vi "Get Menu Items.vi"() -> ()   [LabVIEW 2010]
panel:
  in  "Status 2":string[][](array[string])=[["File: Data Log", "正在进行数据记录"], ["File: Copy Parameters", "正在复制参数"], ["File: Print", "正在打印"], ["File: Export", "正在导出"], ["File: Exit", "退出"], ["Users: Login", "用户登录"], ["Users: Management", "用户管理"], ["System - Comm", "系统通信状态"], ["System: Comm Diags", "系统通信诊断"], ["System: Comm Enable", "通信使能"], ["System: Comm Disable", "通信禁用"], ["System: Snapshot", "系统快照"], ["System: Snapshot Save", "保存快照"], ["System: Snapshot Restore", "恢复快照"], ["System: Snapshot Remove", "删除快照"], ["Recipe: New", "新建Recipe"], ["Recipe: Open", "打开Recipe"], ["Recipe: Save", "保存Recipe"], ["Recipe: Save As", "另存Recipe"], ["Recipe: Remove", "移除Recipe"], ["Recipe: Download", "下载Recipe"], ["Recipe: Calendar", "查看日历"], ["Recipe: Time Builder", "Recipe类型创建器"], ["EventLogs: View", "查看事件记录"], ["EventLogs: Copy To A:", "复制事件记录"], ["EventLogs: Remove", "移除事件记录"], ["TP: Graph", "查看趋势图"], ["TP: Export Graph Data", "导出趋势图数据"], ["View: Alarms", "查看警告"], ["View: F4 Set up", "查看F4设置"], ["Tools: Set F4 Date and Time", "设置F4日期和时间"], ["Tools: F4 Save Change to EE", "保存F4设置"], ["Tools: F4 Profile Control", "F4 Profile控制"], ["Tools: F4 Profile Editor", "F4 Profile编辑器"], ["Help: About", "帮助"]]
  in  "停止":bool=TRUE
  in  "states":string[][](array[string])=[["DAQmx - Clear", "正在清除采集任务"], ["DAQmx - Dynamic  Routine", "正在配置任务"], ["DAQmx - Get Device Info", "正在获得设备信息"], ["DAQmx - Load Settings", "正在加载采集任务"], ["DAQmx - Run", "正在进行采集"], ["DAQmx - Start", "正在启动任务"], ["DAQmx - Tasks Config", "正在配置任务"], ["File - Calibrate", "正在进行通道校准"], ["File - Configure", "正在进行通道配置"], ["Front Pannel - Open", "打开用户面板"], ["Front Pannel - Refresh Display", "更新面板控件 显示"], ["Front Pannel - Set Properties", "设置面板属性"], ["Initialize", "正在进行初始化"], ["No Action", "等待操作中"], ["Operate - Start", "准备试验"], ["Reserve", "保留"], ["Routine - Calibration Dialog", "正在进行通道校准"], ["Routine - Initialize", "正在进行初始化"], ["Routine - Test Header Dialog", "设置试验信息"], ["Users - Login", "用户登录"], ["Users - Login Dialog", "用户登录"], ["Operate - Save Data", "正在进行采集 - 数据保存起始于:"], ["Operate - Static Sample", ""], ["Operate - Query", ""]]
  in  "Status":string[][](array[string])
  in  "menu 2nd order tags":string[][](array[string])
  out "字符串":string
  # "Users: Login\nUsers: Management\nSystem: Comm Enable\nSystem: Comm Disable\nSystem: Comm Diags\nSystem: Snapshot\nSystem: Snapshot Save\nSystem: Snapshot Restore\nSystem: Snapshot Remove\nSystem: Setup Passwords"
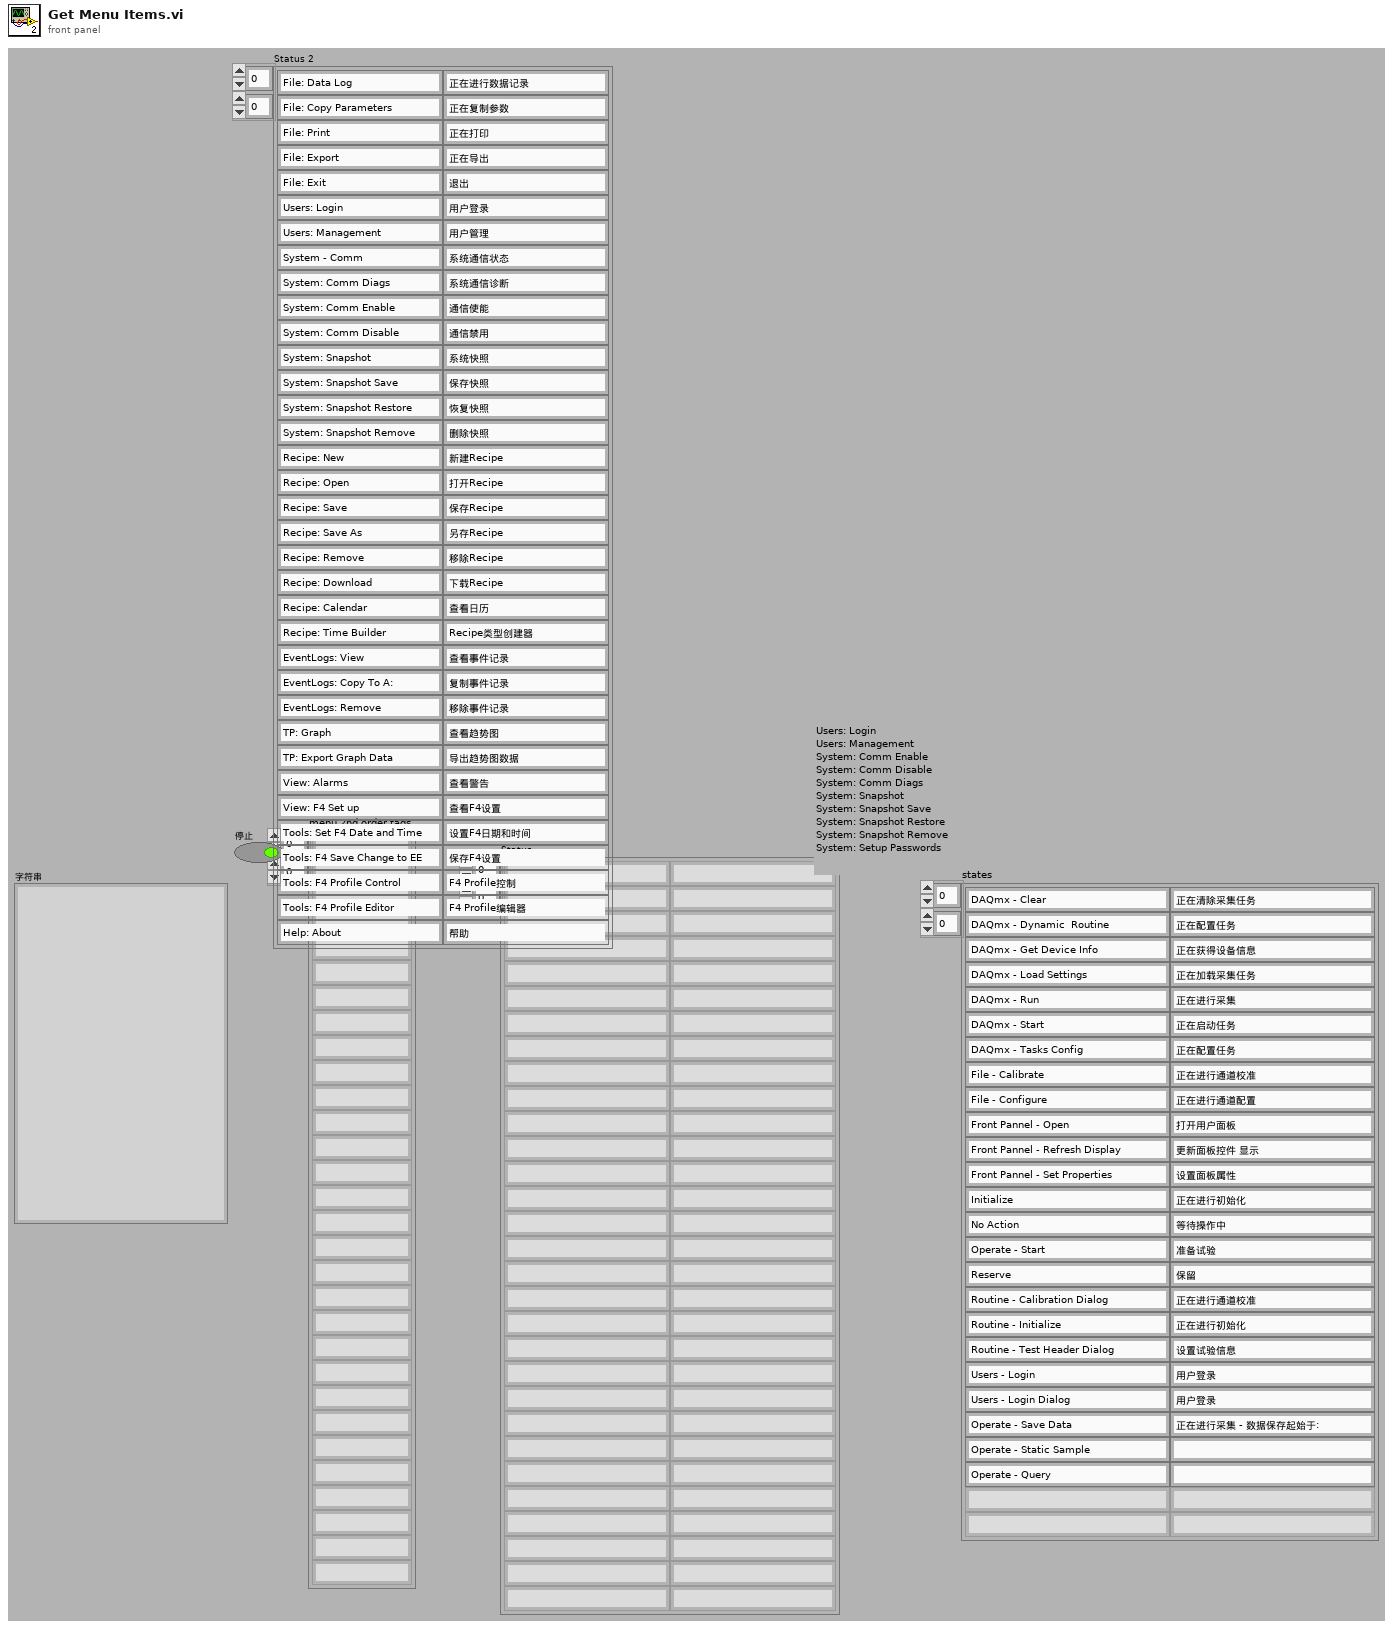
[diagram p1: front panel]
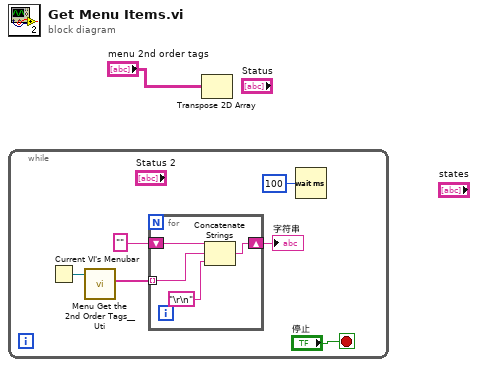
[diagram p0: block diagram]
diagram:
  n1 = while {
    stop <- "停止" stop-if-true
    n2 = Current VI's Menubar() -> (w4:refnum<k9>)
    n3 = call "Menu Get the 2nd Order Tags__Uti.vi"("menu in"=w4) -> ("menu 2nd order tags"=w3:string[])  [unwired: 8 in, 2 out]
    n4 = for {
      shift-right: [w8] -> w2
      shift-left: "" -> [w11]
      tunnel: w3 -> [w10] mode=indexing
      n5 = Concatenate Strings(w11, w10, "\r\n") -> (w8:string)
    }
    "字符串" <- w2
    n6 = Wait (ms)(milliseconds to wait=u32 100 ("等待时间（毫秒）")) -> ()  [unwired: 1 out]
  }
  n7 = Transpose 2D Array(2D array="menu 2nd order tags") -> ()  [unwired: 1 out]
